vi "Remove_Shortcut.vi"(8 "error in (no error)":errorcluster, 10 "index":i32, 11 "Installer in":refnum<class "Installer.lvclass">) -> (0 "error out":errorcluster, 2 "removed shortcut":T1, 3 "Installer out":refnum<class "Installer.lvclass">)   [LabVIEW 2020, in "Installer.lvclass"]
uses:
  <vilib>/AppBuilder/IB_Classes/Installer/Installer.lvclass
  <vilib>/AppBuilder/IB_Classes/Installer/Installer.lvclass/Installer.ctl
  <resource>/Framework/Providers/Builds/Installer/CDK_sTypeDef_ShortcutAddress.ctl
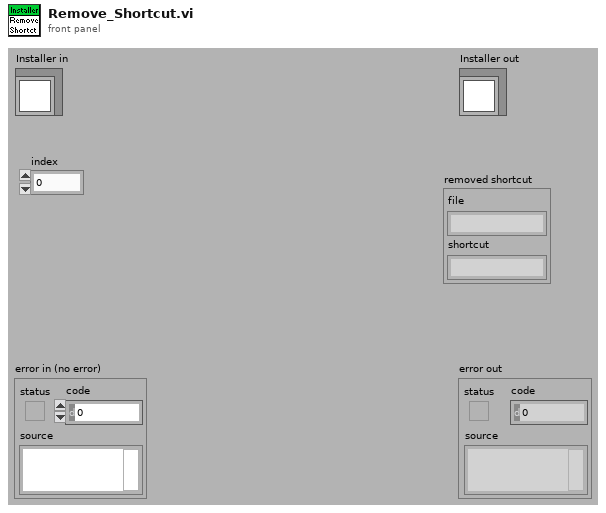
[diagram p1: front panel]
types:
  T1 = typedef "CDK_sTypeDef_ShortcutAddress.ctl" = cluster{"file":string, "shortcut":string}
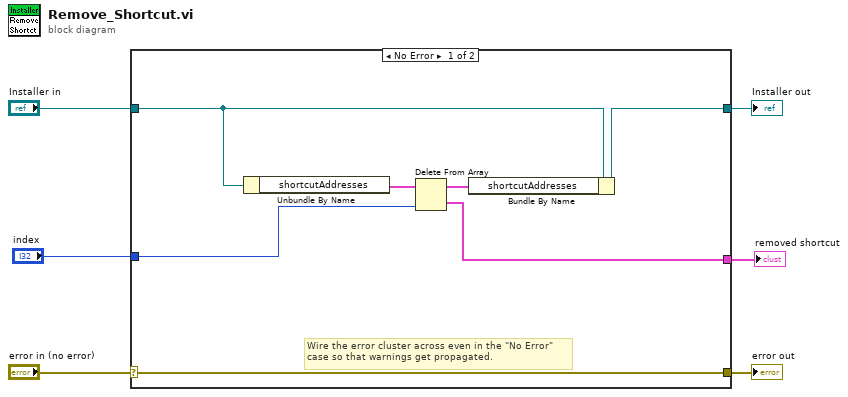
[diagram p0: block diagram]
diagram:
  n1 = case shown="No Error" "error in (no error)" {
    selector: "error in (no error)" -> [w13 w15]
    tunnel: [w13 w15] -> w5
    tunnel: [w9 w14] -> w3
    tunnel: "Installer in" -> [w10 w14]
    tunnel: "index" -> [w8 _]
    tunnel: [w7 _] -> w1
    frame No Error {
      # "Wire the error cluster across even in the \"No Error\"\ncase so that warnings get propagated."
      n2 = Unbundle By Name(w10) -> ("shortcutAddresses"=w12:T1[])
      n3 = Delete From Array(array=w12, index=w8) -> (deleted portion=w7:T1, array with subset deleted=w11:T1[])  [unwired: 1 in]
      n4 = Bundle By Name(cluster=w10, "shortcutAddresses"=w11) -> (w9:refnum<class "Installer.lvclass">)
    }
    frame Error {
    }
  }
  "error out" <- w5
  "Installer out" <- w3
  "removed shortcut" <- w1
